vi "日志、报警信息存储 (子VI).vi"() -> ()   [LabVIEW 2016, in "超标留样集成.lvlib" / "德润DR803L超标留样.lvlib"]
uses:
  <vilib>/ptbypt/NI_PtbyPt.lvlib
panel:
  out "采样器状态":T1
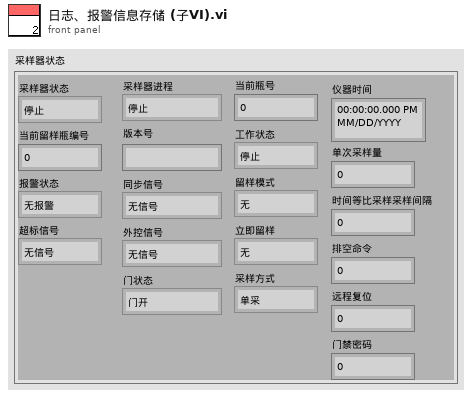
[diagram p1: front panel]
types:
  T1 = cluster{"采样器状态":enum16{"停止", "运行"}, "当前留样瓶编号":u16, "报警状态":enum16{"无报警", "缺水报警"}, "超标信号":enum16{"无信号", "超标信号"}, "采样器进程":enum16{"停止", "待机", "定位校正", "移除瓶盖", "采样瓶排空", "管路润洗", "管存", "进样", "瓶盖密封", "管路排空", "调整采样位置", "采样结束", "采样瓶润洗", "瓶润洗排空"}, "版本号":string, "同步信号":enum16{"无信号", "同步信号"}, "外控信号":enum16{"无信号", "外控信号"}, "门状态":enum16{"门开", "门关"}, "当前瓶号":u16, "工作状态":enum16{"停止", "采样中"}, "留样模式":enum16{"无", "定时留样", "时间等比例", "超标留样", "同步留样", "外控留样"}, "立即留样":enum16{"无", "远程留样"}, "采样方式":enum16{"单采", "双重"}, "仪器时间":timestamp, "单次采样量":u16, "时间等比采样采样间隔":u16, "排空命令":u16, "远程复位":u16, "门禁密码":u16}
  T2 = cluster{"时间标识":timestamp, "设备":string, "日志信息":string}
  T3 = cluster{"时间标识":timestamp, "设备":string, "日志信息":string, "流程参数":string}
  T4 = enum16{"停止", "待机", "定位校正", "移除瓶盖", "采样瓶排空", "管路润洗", "管存", "进样", "瓶盖密封", "管路排空", "调整采样位置", "采样结束", "采样瓶润洗", "瓶润洗排空"}
  T5 = enum16{"无", "定时留样", "时间等比例", "超标留样", "同步留样", "外控留样"}
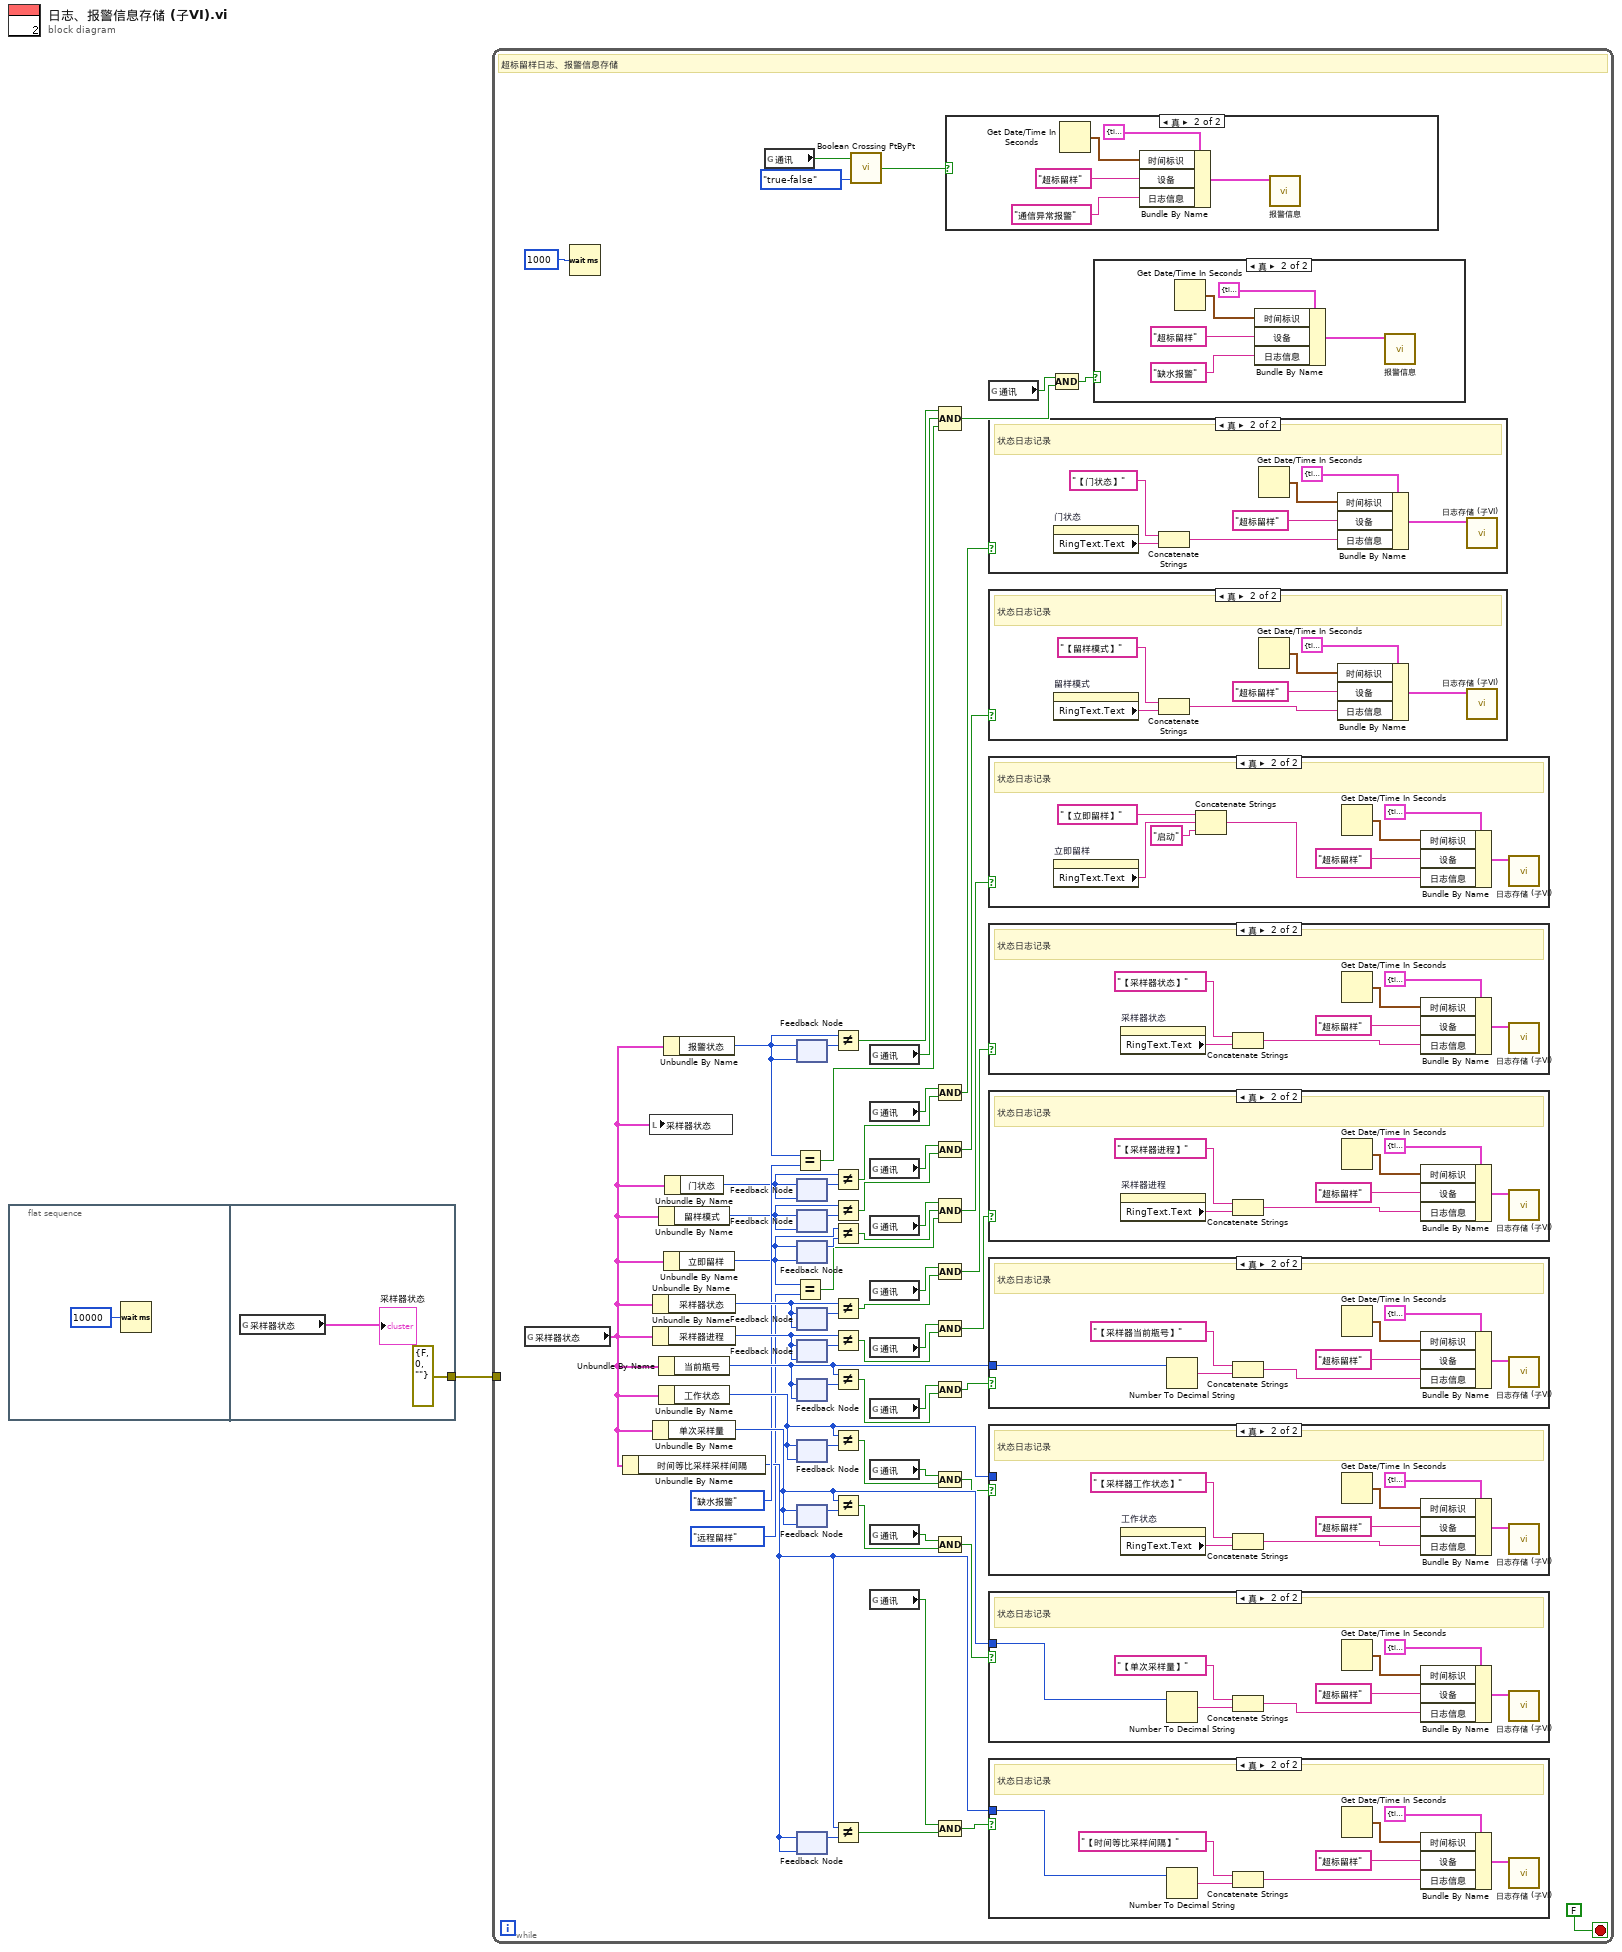
[diagram p0: block diagram]
diagram:
  n1 = flat-sequence {
    tunnel: [errorcluster {"status"=FALSE, "code"=0, "source"=""} ("错误常量")] -> w1
    frame #0 {
      n2 = Wait (ms)(milliseconds to wait=u32 10000 ("等待时间（毫秒）")) -> ()  [unwired: 1 out]
    }
    frame #1 {
      n3 = global read "超标留样全局.vi" "采样器状态"() -> (→"采样器状态":T1)
    }
  }
  n4 = while {
    tunnel: w1 -> [_]
    stop <- FALSE stop-if-true
    # "超标留样日志、报警信息存储"
    n5 = global read "超标留样全局.vi" "采样器状态"() -> (w8:T1)
    n6 = Wait (ms)(milliseconds to wait=u32 1000 ("等待时间（毫秒）")) -> ()  [unwired: 1 out]
    n7 = Unbundle By Name(w8) -> ("时间等比采样采样间隔"=w44:u16)
    n8 = local write "采样器状态"(w8) -> ()
    n9 = Unbundle By Name(w8) -> ("采样器状态"=w63:enum16{"停止", "运行"})
    n10 = Unbundle By Name(w8) -> ("采样器进程"=w62:T4)
    n11 = Unbundle By Name(w8) -> ("单次采样量"=w55:u16)
    n12 = Unbundle By Name(w8) -> ("留样模式"=w47:T5)
    n13 = Unbundle By Name(w8) -> ("当前瓶号"=w59:u16)
    n14 = Unbundle By Name(w8) -> ("工作状态"=w58:enum16{"停止", "采样中"})
    n15 = Unbundle By Name(w8) -> ("报警状态"=w50:enum16{"无报警", "缺水报警"})
    n16 = Unbundle By Name(w8) -> ("立即留样"=w43:enum16{"无", "远程留样"})
    n17 = Unbundle By Name(w8) -> ("门状态"=w48:enum16{"门开", "门关"})
    n18 = global read "超标留样全局.vi" "通讯"() -> (w7:bool)
    n19 = Equal?(x=w50, y=enum16{"无报警", "缺水报警"}."缺水报警" ("报警状态")) -> (x = y?=w38:bool)
    n20 = Equal?(x=w43, y=enum16{"无", "远程留样"}."远程留样" ("立即留样")) -> (x = y?=w11:bool)
    n21 = feedback #1(w50) -> (w53:enum16{"无报警", "缺水报警"})
    n22 = feedback-in #1(w50) -> ()
    n23 = feedback #2(w48) -> (w49:enum16{"门开", "门关"})
    n24 = feedback-in #2(w48) -> ()
    n25 = feedback #3(w47) -> (w46:T5)
    n26 = feedback-in #3(w47) -> ()
    n27 = feedback #4(w43) -> (w42:enum16{"无", "远程留样"})
    n28 = feedback-in #4(w43) -> ()
    n29 = feedback #5(w63) -> (w64:enum16{"停止", "运行"})
    n30 = feedback-in #5(w63) -> ()
    n31 = feedback #6(w62) -> (w61:T4)
    n32 = feedback-in #6(w62) -> ()
    n33 = feedback #7(w59) -> (w60:u16)
    n34 = feedback-in #7(w59) -> ()
    n35 = feedback #8(w58) -> (w57:enum16{"停止", "采样中"})
    n36 = feedback-in #8(w58) -> ()
    n37 = feedback #9(w55) -> (w56:u16)
    n38 = feedback-in #9(w55) -> ()
    n39 = feedback #10(w44) -> (w45:u16)
    n40 = feedback-in #10(w44) -> ()
    n41 = Not Equal?(x=w50, y=w53) -> (x != y?=w37:bool)
    n42 = Not Equal?(x=w48, y=w49) -> (x != y?=w34:bool)
    n43 = Not Equal?(x=w47, y=w46) -> (x != y?=w26:bool)
    n44 = Not Equal?(x=w43, y=w42) -> (x != y?=w10:bool)
    n45 = Not Equal?(x=w63, y=w64) -> (x != y?=w28:bool)
    n46 = Not Equal?(x=w62, y=w61) -> (x != y?=w29:bool)
    n47 = Not Equal?(x=w59, y=w60) -> (x != y?=w22:bool)
    n48 = Not Equal?(x=w58, y=w57) -> (x != y?=w20:bool)
    n49 = Not Equal?(x=w55, y=w56) -> (x != y?=w17:bool)
    n50 = Not Equal?(x=w44, y=w45) -> (x != y?=w13:bool)
    n51 = call <vilib>:"Boolean Crossing PtByPt.vi"("direction"=enum16{"either", "false-true", "true-false"}."true-false", "input"=w7) -> ("crossing"=w5:bool)  [unwired: 1 in]
    n52 = global read "超标留样全局.vi" "通讯"() -> (w40:bool)
    n53 = global read "超标留样全局.vi" "通讯"() -> (w36:bool)
    n54 = global read "超标留样全局.vi" "通讯"() -> (w33:bool)
    n55 = global read "超标留样全局.vi" "通讯"() -> (w12:bool)
    n56 = global read "超标留样全局.vi" "通讯"() -> (w32:bool)
    n57 = global read "超标留样全局.vi" "通讯"() -> (w31:bool)
    n58 = global read "超标留样全局.vi" "通讯"() -> (w24:bool)
    n59 = global read "超标留样全局.vi" "通讯"() -> (w21:bool)
    n60 = global read "超标留样全局.vi" "通讯"() -> (w18:bool)
    n61 = global read "超标留样全局.vi" "通讯"() -> (w15:bool)
    n62 = Compound Arithmetic op=AND ("复合运算")(w37, w40, w38) -> (w39:bool)
    n63 = Compound Arithmetic op=AND ("复合运算")(w36, w34) -> (w35:bool)
    n64 = Compound Arithmetic op=AND ("复合运算")(w33, w26) -> (w25:bool)
    n65 = Compound Arithmetic op=AND ("复合运算")(w12, w10, w11) -> (w9:bool)
    n66 = Compound Arithmetic op=AND ("复合运算")(w32, w28) -> (w27:bool)
    n67 = Compound Arithmetic op=AND ("复合运算")(w31, w29) -> (w30:bool)
    n68 = Compound Arithmetic op=AND ("复合运算")(w24, w22) -> (w23:bool)
    n69 = Compound Arithmetic op=AND ("复合运算")(w21, w20) -> (w19:bool)
    n70 = Compound Arithmetic op=AND ("复合运算")(w18, w17) -> (w16:bool)
    n71 = Compound Arithmetic op=AND ("复合运算")(w15, w13) -> (w14:bool)
    n72 = case shown="真" w5 {
      frame False {
      }
      frame True {
        n73 = Get Date/Time In Seconds() -> (seconds since 1Jan1904=w67:timestamp)
        n74 = Bundle By Name(cluster=T2 {"时间标识"=timestamp(0 s since 1904-01-01), "设备"="", "日志信息"=""} ("data in"), "时间标识"=w67, "设备"="超标留样", "日志信息"="通信异常报警") -> (w71:T2)
        n75 = call "报警信息.vi"("data in"=w71) -> ()  [unwired: 10 in, 1 out]
      }
    }
    n76 = global read "超标留样全局.vi" "通讯"() -> (w54:bool)
    n77 = case shown="真" w35 {
      frame False {
      }
      frame True {
        # "状态日志记录"
        n78 = property on="门状态" class="Enum (严格)"() -> ("RingText.Text"=w95:string)  [unwired: 2 in, 2 out]
        n79 = Concatenate Strings("【门状态】" ("日志信息"), w95) -> (w101:string)
        n80 = Get Date/Time In Seconds() -> (seconds since 1Jan1904=w98:timestamp)
        n81 = Bundle By Name(cluster=T3 {"时间标识"=timestamp(0 s since 1904-01-01), "设备"="", "日志信息"="", "流程参数"=""} ("data in"), "时间标识"=w98, "设备"="超标留样", "日志信息"=w101) -> (w97:T3)
        n82 = call "日志存储 (子VI).vi"("data in"=w97) -> ()  [unwired: 11 in]
      }
    }
    n83 = case shown="真" w25 {
      frame False {
      }
      frame True {
        # "状态日志记录"
        n84 = property on="留样模式" class="Enum (严格)"() -> ("RingText.Text"=w88:string)  [unwired: 2 in, 2 out]
        n85 = Concatenate Strings("【留样模式】" ("日志信息"), w88) -> (w94:string)
        n86 = Get Date/Time In Seconds() -> (seconds since 1Jan1904=w91:timestamp)
        n87 = Bundle By Name(cluster=T3 {"时间标识"=timestamp(0 s since 1904-01-01), "设备"="", "日志信息"="", "流程参数"=""} ("data in"), "时间标识"=w91, "设备"="超标留样", "日志信息"=w94) -> (w90:T3)
        n88 = call "日志存储 (子VI).vi"("data in"=w90) -> ()  [unwired: 11 in]
      }
    }
    n89 = case shown="真" w9 {
      frame False {
      }
      frame True {
        # "状态日志记录"
        n90 = property on="立即留样" class="Enum (严格)"() -> ("RingText.Text"=w73:string)  [unwired: 2 in, 2 out]
        n91 = Concatenate Strings("【立即留样】" ("日志信息"), w73, "启动" ("字符串")) -> (w79:string)
        n92 = Get Date/Time In Seconds() -> (seconds since 1Jan1904=w76:timestamp)
        n93 = Bundle By Name(cluster=T3 {"时间标识"=timestamp(0 s since 1904-01-01), "设备"="", "日志信息"="", "流程参数"=""} ("data in"), "时间标识"=w76, "设备"="超标留样", "日志信息"=w79) -> (w75:T3)
        n94 = call "日志存储 (子VI).vi"("data in"=w75) -> ()  [unwired: 11 in]
      }
    }
    n95 = case shown="真" w27 {
      frame False {
      }
      frame True {
        # "状态日志记录"
        n96 = property on="采样器状态" class="Enum (严格)"() -> ("RingText.Text"=w137:string)  [unwired: 2 in, 2 out]
        n97 = Concatenate Strings("【采样器状态】" ("日志信息"), w137) -> (w143:string)
        n98 = Get Date/Time In Seconds() -> (seconds since 1Jan1904=w140:timestamp)
        n99 = Bundle By Name(cluster=T3 {"时间标识"=timestamp(0 s since 1904-01-01), "设备"="", "日志信息"="", "流程参数"=""} ("data in"), "时间标识"=w140, "设备"="超标留样", "日志信息"=w143) -> (w139:T3)
        n100 = call "日志存储 (子VI).vi"("data in"=w139) -> ()  [unwired: 11 in]
      }
    }
    n101 = case shown="真" w30 {
      frame False {
      }
      frame True {
        # "状态日志记录"
        n102 = property on="采样器进程" class="Enum (严格)"() -> ("RingText.Text"=w130:string)  [unwired: 2 in, 2 out]
        n103 = Concatenate Strings("【采样器进程】" ("日志信息"), w130) -> (w136:string)
        n104 = Get Date/Time In Seconds() -> (seconds since 1Jan1904=w133:timestamp)
        n105 = Bundle By Name(cluster=T3 {"时间标识"=timestamp(0 s since 1904-01-01), "设备"="", "日志信息"="", "流程参数"=""} ("data in"), "时间标识"=w133, "设备"="超标留样", "日志信息"=w136) -> (w132:T3)
        n106 = call "日志存储 (子VI).vi"("data in"=w132) -> ()  [unwired: 11 in]
      }
    }
    n107 = case shown="真" w23 {
      tunnel: w59 -> [_ w123]
      frame False {
      }
      frame True {
        # "状态日志记录"
        n108 = Number To Decimal String(number=w123) -> (decimal integer string=w122:string)  [unwired: 1 in]
        n109 = Concatenate Strings("【采样器当前瓶号】" ("日志信息"), w122) -> (w129:string)
        n110 = Get Date/Time In Seconds() -> (seconds since 1Jan1904=w126:timestamp)
        n111 = Bundle By Name(cluster=T3 {"时间标识"=timestamp(0 s since 1904-01-01), "设备"="", "日志信息"="", "流程参数"=""} ("data in"), "时间标识"=w126, "设备"="超标留样", "日志信息"=w129) -> (w125:T3)
        n112 = call "日志存储 (子VI).vi"("data in"=w125) -> ()  [unwired: 11 in]
      }
    }
    n113 = case shown="真" w19 {
      tunnel: w58 -> [_ _]
      frame False {
      }
      frame True {
        # "状态日志记录"
        n114 = property on="工作状态" class="Enum (严格)"() -> ("RingText.Text"=w115:string)  [unwired: 2 in, 2 out]
        n115 = Concatenate Strings("【采样器工作状态】" ("日志信息"), w115) -> (w121:string)
        n116 = Get Date/Time In Seconds() -> (seconds since 1Jan1904=w118:timestamp)
        n117 = Bundle By Name(cluster=T3 {"时间标识"=timestamp(0 s since 1904-01-01), "设备"="", "日志信息"="", "流程参数"=""} ("data in"), "时间标识"=w118, "设备"="超标留样", "日志信息"=w121) -> (w117:T3)
        n118 = call "日志存储 (子VI).vi"("data in"=w117) -> ()  [unwired: 11 in]
      }
    }
    n119 = case shown="真" w16 {
      tunnel: w55 -> [_ w108]
      frame False {
      }
      frame True {
        # "状态日志记录"
        n120 = Number To Decimal String(number=w108) -> (decimal integer string=w107:string)  [unwired: 1 in]
        n121 = Concatenate Strings("【单次采样量】" ("日志信息"), w107) -> (w114:string)
        n122 = Get Date/Time In Seconds() -> (seconds since 1Jan1904=w111:timestamp)
        n123 = Bundle By Name(cluster=T3 {"时间标识"=timestamp(0 s since 1904-01-01), "设备"="", "日志信息"="", "流程参数"=""} ("data in"), "时间标识"=w111, "设备"="超标留样", "日志信息"=w114) -> (w110:T3)
        n124 = call "日志存储 (子VI).vi"("data in"=w110) -> ()  [unwired: 11 in]
      }
    }
    n125 = case shown="真" w14 {
      tunnel: w44 -> [_ w81]
      frame False {
      }
      frame True {
        # "状态日志记录"
        n126 = Number To Decimal String(number=w81) -> (decimal integer string=w80:string)  [unwired: 1 in]
        n127 = Concatenate Strings("【时间等比采样间隔】" ("日志信息"), w80) -> (w87:string)
        n128 = Get Date/Time In Seconds() -> (seconds since 1Jan1904=w84:timestamp)
        n129 = Bundle By Name(cluster=T3 {"时间标识"=timestamp(0 s since 1904-01-01), "设备"="", "日志信息"="", "流程参数"=""} ("data in"), "时间标识"=w84, "设备"="超标留样", "日志信息"=w87) -> (w83:T3)
        n130 = call "日志存储 (子VI).vi"("data in"=w83) -> ()  [unwired: 11 in]
      }
    }
    n131 = Compound Arithmetic op=AND ("复合运算")(w54, w39) -> (w52:bool)
    n132 = case shown="真" w52 {
      frame False {
      }
      frame True {
        n133 = Get Date/Time In Seconds() -> (seconds since 1Jan1904=w106:timestamp)
        n134 = Bundle By Name(cluster=T2 {"时间标识"=timestamp(0 s since 1904-01-01), "设备"="", "日志信息"=""} ("data in"), "时间标识"=w106, "设备"="超标留样", "日志信息"="缺水报警") -> (w102:T2)
        n135 = call "报警信息.vi"("data in"=w102) -> ()  [unwired: 10 in, 1 out]
      }
    }
  }
